vi "FRCts20_WebMethods_Convert_Request.vi"(8 "error in (no error)":errorcluster, 10 "Team Out":T8, 11 "Request Out":T9) -> (0 "error out":errorcluster, 3 "Request+Team":cluster{"Request":T1, "Team":T4})   [LabVIEW 2012, in "FRCts20_WebMethods.lvlib"]
uses:
  FRCts20_WebMethods.lvlib
  Backend/source/VI Source/FRCts20_Backend_API/FRCts20_Backend_API_Request.ctl
  Backend/source/VI Source/FRCts20_Backend_API/FRCts20_Backend_API_Status.ctl
  Backend/source/VI Source/FRCts20_Backend_API/FRCts20_Backend_API_Team.ctl
  Backend/source/VI Source/FRCts20_Backend_API/FRCts20_Backend_API_SW.ctl
  ESP Engine/source/VI Source/TypeDefs/FRCts20_EspEngine_Request.ctl
  Web Method Public Interface/FRCts20_WebMethods_ctl_request.ctl
  ESP Engine/source/VI Source/TypeDefs/FRCts20_EspEngine_Team.ctl
  Web Method Public Interface/FRCts20_WebMethods_ctl_singleTeam.ctl
  Web Method Public Interface/FRCts20_WebMethods_ctl_teamIdentifier.ctl
  Backend/source/VI Source/FRCts20_Backend_API/FRCts20_Backend_API.lvlib
  ESP Engine/source/VI Source/FRCts20_EspEngine.lvlib
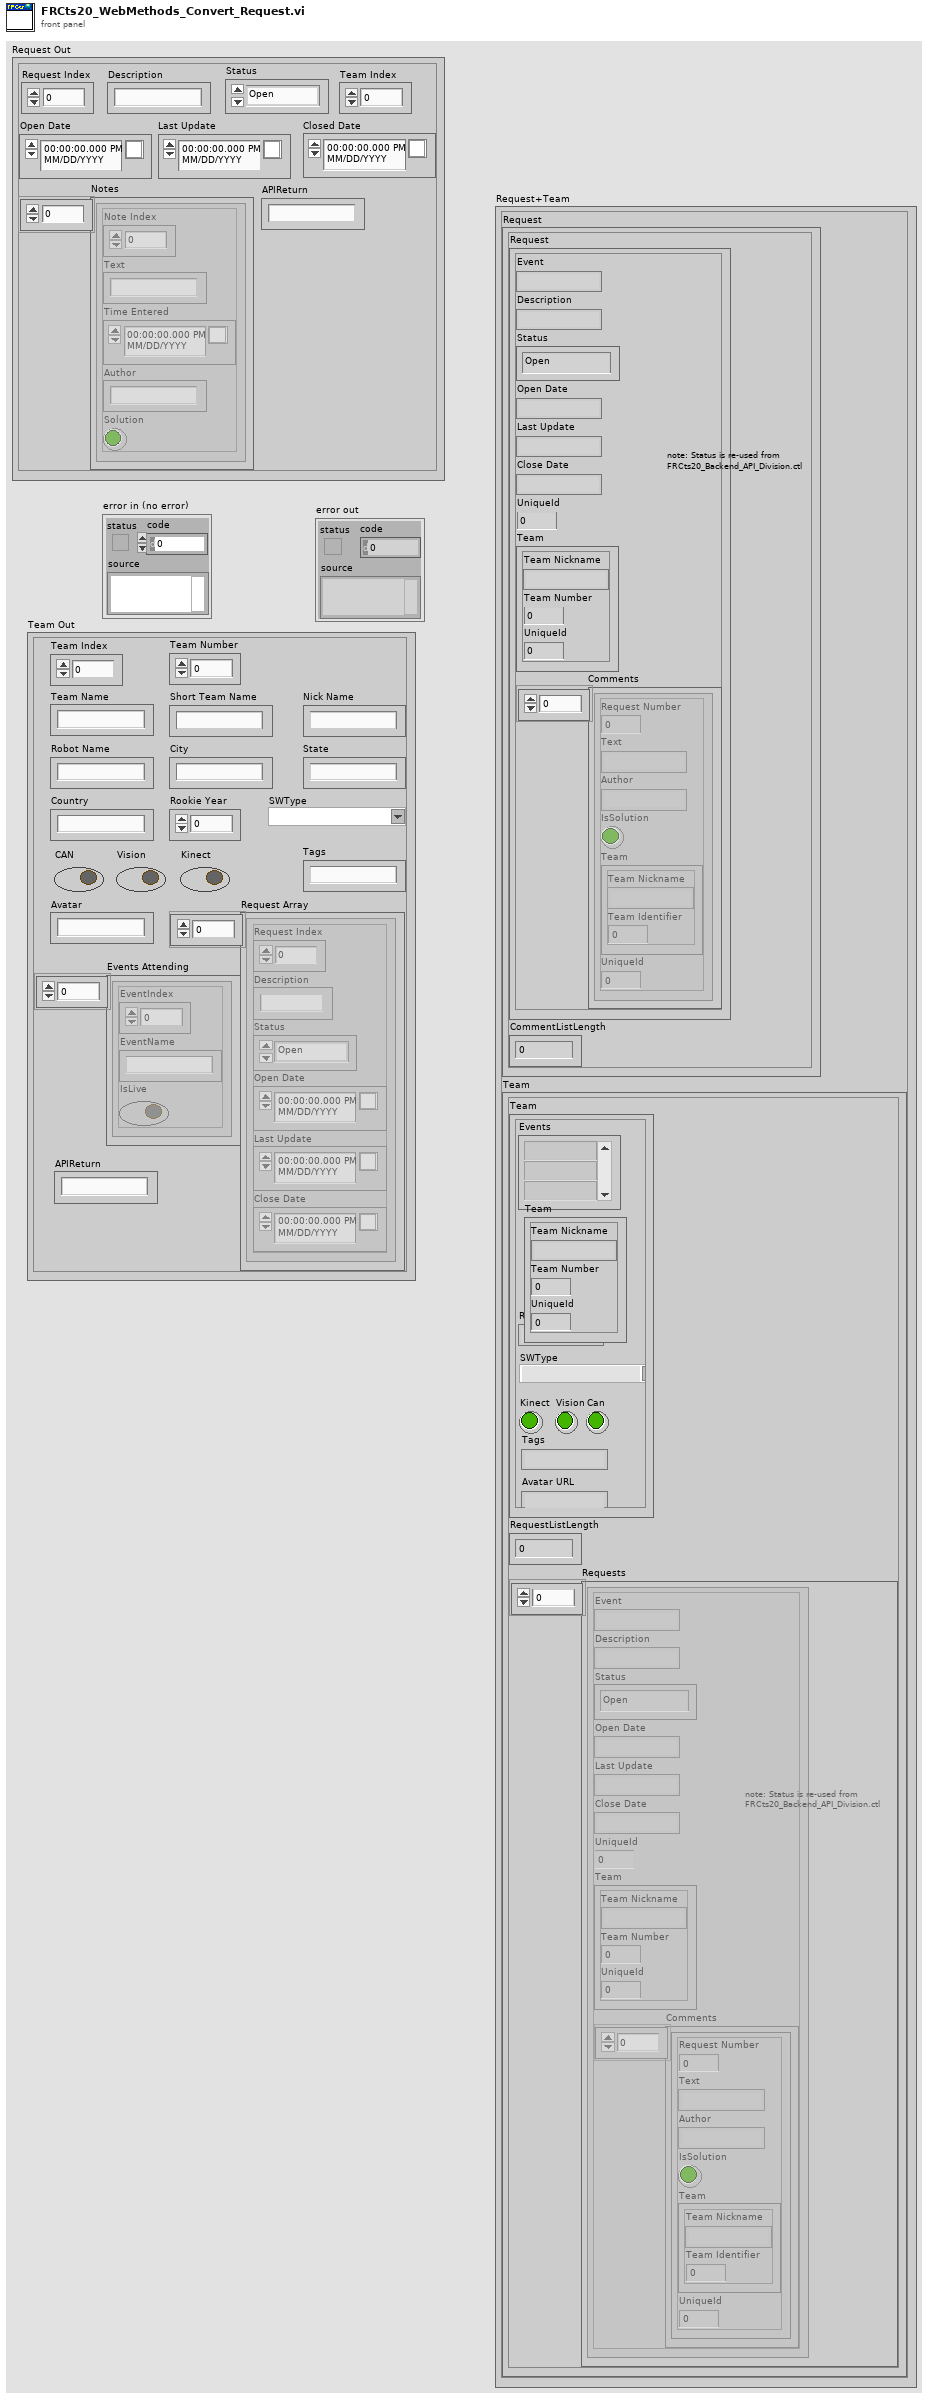
[diagram p1: front panel]
types:
  T1 = typedef "FRCts20_EspEngine.lvlib/FRCts20_EspEngine_Request.ctl" = cluster{"Request":T2, "CommentListLength":i16}
  T2 = typedef "FRCts20_WebMethods.lvlib/FRCts20_WebMethods_ctl_request.ctl" = cluster{"Event":string, "Description":string, "Status":T3, "Open Date":string, "Last Update":string, "Close Date":string, "UniqueId":i32, "Team":cluster{"Team Nickname":string, "Team Number ":i32, "UniqueId":i32}, "Comments":cluster{"Request Number":dbl, "Text":string, "Author":string, "IsSolution":bool, "Team":cluster{"Team Nickname":string, "Team Identifier ":dbl}, "UniqueId":i32}[]}
  T3 = typedef "FRCts20_Backend_API.lvlib/FRCts20_Backend_API_Status.ctl" = enum16{"Open", "In Work", "Closed"}
  T4 = typedef "FRCts20_EspEngine.lvlib/FRCts20_EspEngine_Team.ctl" = cluster{"Team":T5, "RequestListLength":i16, "Requests":T2[]}
  T5 = typedef "FRCts20_WebMethods.lvlib/FRCts20_WebMethods_ctl_singleTeam.ctl" = cluster{"Events":string[], "Robot Name":string, "Kinect":bool, "Vision":bool, "Can":bool, "Tags":string, "Avatar URL":string, "Team":T6, "SWType":T7}
  T6 = typedef "FRCts20_WebMethods.lvlib/FRCts20_WebMethods_ctl_teamIdentifier.ctl" = cluster{"Team Nickname":string, "Team Number ":u32, "UniqueId":u32}
  T7 = typedef "FRCts20_Backend_API.lvlib/FRCts20_Backend_API_SW.ctl" = string
  T8 = typedef "FRCts20_Backend_API.lvlib/FRCts20_Backend_API_Team.ctl" = cluster{"Team Index":u32, "Team Number":u32, "Team Name":string, "Short Team Name":string, "Nick Name":string, "Robot Name":string, "City":string, "State":string, "Country":string, "Rookie Year":u32, "SWType":T7, "CAN":bool, "Vision":bool, "Kinect":bool, "Tags":string, "Avatar":string, "Request Array":cluster{"Request Index":u32, "Description":string, "Status":T3, "Open Date":timestamp, "Last Update":timestamp, "Close Date":timestamp}[], "Events Attending":cluster{"EventIndex":dbl, "EventName":string, "IsLive":bool}[], "APIReturn":string}
  T9 = typedef "FRCts20_Backend_API.lvlib/FRCts20_Backend_API_Request.ctl" = cluster{"Request Index":u32, "Description":string, "Status":T3, "Open Date":timestamp, "Last Update":timestamp, "Closed Date":timestamp, "Notes":cluster{"Note Index":u32, "Text":string, "Time Entered":timestamp, "Author":string, "Solution":bool}[], "Team Index":u32, "APIReturn":string}
  T10 = cluster{"Request Number":dbl, "Text":string, "Author":string, "IsSolution":bool, "Team":cluster{"Team Nickname":string, "Team Identifier ":dbl}, "UniqueId":i32}
  T11 = cluster{"Request Index":u32, "Description":string, "Status":T3, "Open Date":timestamp, "Last Update":timestamp, "Close Date":timestamp}[]
  T12 = cluster{"Note Index":u32, "Text":string, "Time Entered":timestamp, "Author":string, "Solution":bool}[]
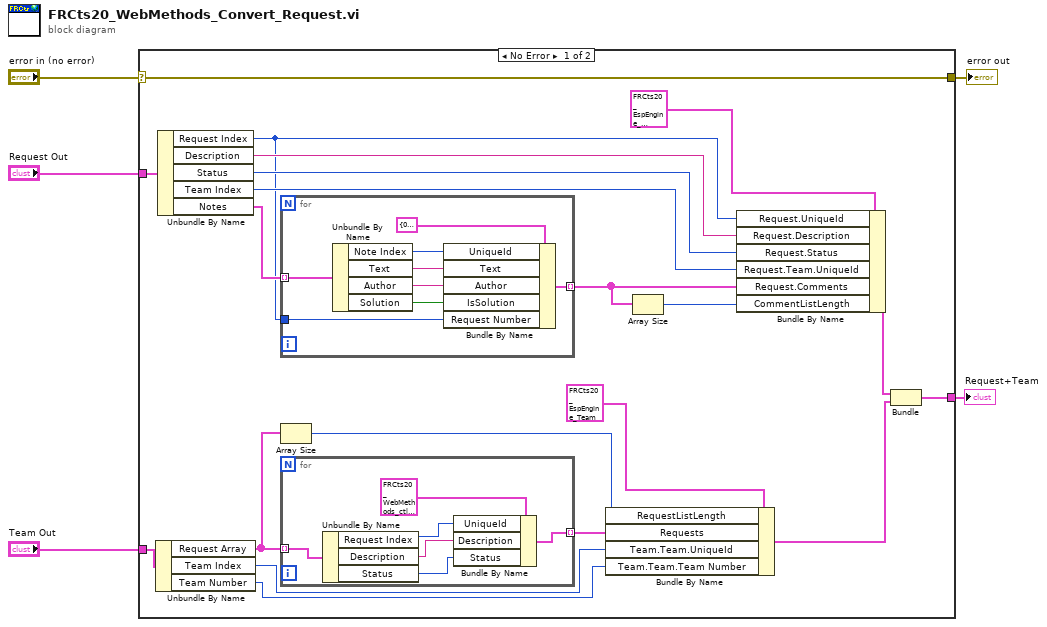
[diagram p0: block diagram]
diagram:
  n1 = case shown="No Error" "error in (no error)" {
    selector: "error in (no error)" -> [w16 w40]
    tunnel: [w16 w40] -> w5
    tunnel: "Request Out" -> [w17 _]
    tunnel: "Team Out" -> [w14 _]
    tunnel: [w8 _] -> w1
    frame No Error {
      n2 = Unbundle By Name(w14) -> ("Request Array"=w12:T11, "Team Index"=w7:u32, "Team Number"=w6:u32)
      n3 = Unbundle By Name(w17) -> ("Request Index"=w20:u32, "Description"=w24:string, "Status"=w23:T3, "Team Index"=w22:u32, "Notes"=w21:T12)
      n4 = for {
        tunnel: [w38] -> w18 mode=indexing
        tunnel: w21 -> [w37] mode=indexing
        tunnel: w20 -> [w32]
        n5 = Unbundle By Name(w37) -> ("Note Index"=w36:u32, "Text"=w35:string, "Author"=w34:string, "Solution"=w33:bool)
        n6 = Bundle By Name(cluster=T10 {"Request Number"=0.0, "Text"="", "Author"="", "IsSolution"=FALSE, "Team"={"Team Nickname"="", "Team Identifier "=0.0}, "UniqueId"=0} ("Comment"), "UniqueId"=w36, "Text"=w35, "Author"=w34, "IsSolution"=w33, "Request Number"=w32) -> (w38:T10)
      }
      n7 = Array Size(array=w12) -> (size(s)=w13:i32)
      n8 = for {
        tunnel: w12 -> [w31] mode=indexing
        tunnel: [w27] -> w11 mode=indexing
        n9 = Unbundle By Name(w31) -> ("Request Index"=w29:u32, "Description"=w28:string, "Status"=w26:T3)
        n10 = Bundle By Name(cluster=T2 {"Event"="", "Description"="", "Status"=enum."Open", "Open Date"="", "Last Update"="", "Close Date"="", "UniqueId"=0, "Team"={"Team Nickname"="", "Team Number "=0, "UniqueId"=0}, "Comments"=[]} ("Request"), "UniqueId"=w29, "Description"=w28, "Status"=w26) -> (w27:T2)
      }
      n11 = Bundle By Name(cluster=T4 {"Team"={"Events"=[], "Robot Name"="", "Kinect"=FALSE, "Vision"=FALSE, "Can"=FALSE, "Tags"="", "Avatar URL"="", "Team"={"Team Nickname"="", "Team Number "=0, "UniqueId"=0}, "SWType"=""}, "RequestListLength"=0, "Requests"=[]} ("Team"), "RequestListLength"=w13, "Requests"=w11, "Team.Team.UniqueId"=w7, "Team.Team.Team Number"=w6) -> (w9:T4)
      n12 = Array Size(array=w18) -> (size(s)=w19:i32)
      n13 = Bundle By Name(cluster=T1 {"Request"={"Event"="", "Description"="", "Status"=enum."Open", "Open Date"="", "Last Update"="", "Close Date"="", "UniqueId"=0, "Team"={"Team Nickname"="", "Team Number "=0, "UniqueId"=0}, "Comments"=[]}, "CommentListLength"=0} ("Request"), "Request.UniqueId"=w20, "Request.Description"=w24, "Request.Status"=w23, "Request.Team.UniqueId"=w22, "Request.Comments"=w18, "CommentListLength"=w19) -> (w10:T1)
      n14 = Bundle("Request"=w10, "Team"=w9) -> (w8:cluster{"Request":T1, "Team":T4})  [unwired: 1 in]
    }
    frame Error {
    }
  }
  "error out" <- w5
  "Request+Team" <- w1
